vi "PH_Beamline.Calc Booster State.vi"(0 "i ref in":refnum<vi>, 2 "PA Exit closed or shining into LL":bool, 5 "error in (no error)":errorcluster) -> (14 "i ref out":refnum<vi>, 16 "Not shining to Mirrortower":bool, 17 "Not shining Experiment LB":bool, 19 "error out":errorcluster)   [LabVIEW 2014, in "PH_Beamline.lvlib"]
doc: "This VI calculates the Booster state of the Beamline."
uses:
  PH_Beamline.lvlib
  PH_Common/PH_Common.lvlib
  PH_BL-Master/PH_BL-Master.lvlib
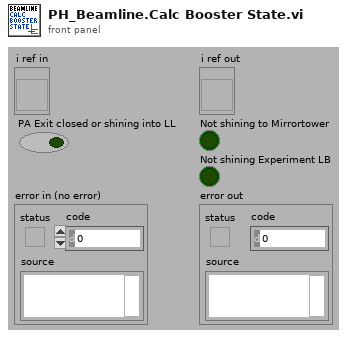
[diagram p1: front panel]
types:
  T1 = typedef "PH_Beamline.lvlib/PH_Beamline.i attribute.ctl" = cluster{"GUI Refs":cluster{"PA ok":refnum<vi>, "MA ok":refnum<vi>, "fs FE ok":refnum<vi>, "ns FE ok":refnum<vi>, "PA ED ok":refnum<vi>, "MAS ok":refnum<vi>, "Booster ok":refnum<vi>, "Mirrortower ok":refnum<vi>, "In.-Box ok":refnum<vi>, "Compressor ok":refnum<vi>, "Experiment LB ok":refnum<vi>, "Experiment LL ok":refnum<vi>, "PHELIX_Beckhoff_Watchdog":refnum<vi>, "Shutters closed":refnum<vi>, "uOPA ok":refnum<vi>, "Vacuum no shotcond Comp LB":refnum<vi>}, "Refs BL MA":refnum<vi>[], "Refs BL MA-IB":refnum<vi>[], "Refs BL fs":refnum<vi>[], "Refs BL PA ED":refnum<vi>[], "Refs BL MAS":refnum<vi>[], "Refs BL Boo":refnum<vi>[], "Refs BL ns":refnum<vi>[], "Refs BL Mirrortower":refnum<vi>[], "Refs BL Compressor":refnum<vi>[], "Refs BL Exp LB":refnum<vi>[], "Radiation Safety":cluster{"Exp Laserbay":cluster{"Ref Op Mode":refnum<vi>, "Ref Laserbay evacuated":refnum<vi>, "Tagname LB evacuated":string, "Shot Mode":T2, "Laserbay evacuated?":i32, "Tagname HV room locked":string, "HV room locked?":i32, "Ref HV room locked":refnum<vi>, "Tagname bridged?":string, "Ref Bridge":refnum<vi>, "I<1E18W/cm²":bool}, "Exp Laserlab":cluster{"Ref Op Mode":refnum<vi>, "Ref Laserlab evacuated":refnum<vi>, "Tagname LL evacuated":string, "Shot Mode":T2, "Laserlab evacuated?":i32, "Tagname bridged?":string, "Ref Bridge":refnum<vi>, "I<1E18W/cm²":bool}}, "Refs BL LL":refnum<vi>[], "PP Igni Heating GUI Refs":refnum<vi>[], "PP Igni Heating Tagnames ":string[], "Refs BL PA":cluster{"undelayed Line before Shutter":refnum<vi>[], "undelayed Line after Shutter":refnum<vi>[], "before Bypass":refnum<vi>[], "delayed Line before Shutter":refnum<vi>[], "delayed Line after Shutter":refnum<vi>[], "before Shutter Input":refnum<vi>[], "after Shutter Input":refnum<vi>[], "Bypass":refnum<vi>[], "before Shutter Exit":refnum<vi>[], "after Shutter Exit":refnum<vi>[], "to MA":refnum<vi>[], "to Lab":refnum<vi>[]}, "BL":cluster{"YLF_BL_Status":i32, "fs_BL_Status":i32, "fs_YLF_BL_Status":i32, "ns_BL_Status":i32, "PA_Input_BL_Status":i32, "PA_UnDelay_BL_Status":i32, "PA_Delay_BL_Status":i32, "PA_BL_Status":i32, "PA_Bypass_BL_Status":i32, "PA_Exit_BL_Status":i32, "PA_LL_BL_Status":i32, "LL_BL_Status":i32, "PA_MA_BL_Status":i32, "MA_Exit_BL_Status":i32, "MA_Z6_BL_Status":i32, "Z6_BL_Status":i32, "MA_LB_BL_Status":i32, "LB_TB2_BL_Status":i32, "PA_before_Bypass_BL_Status":i32, "LB_TB3_BL_Status":i32}, "State Subsystems":cluster{"PA":bool, "MA":bool, "ns FE":bool, "fs FE":bool, "PA ED":bool, "In.-Box":bool, "MAS":bool, "Booster":bool, "Mirrortower":bool, "Compressor":bool, "Experiment LB":bool, "Experiment LL":bool, "uOPA":bool}, "Status Subscriber Information":T3, "Refs BL uOPA":refnum<vi>[], "PA_Input_2_Beam_6PWpGUI not linked?":bool, "PA_Input_Delay_6PGUI not linked?":bool, "Settings":T6}
  T2 = typedef "PH_Beamline.lvlib/PH_Beamline.Operation Mode.ctl" = i32
  T3 = typedef "PH_Beamline.lvlib/PH_Beamline.Status Subscriber Information.ctl" = cluster{"fs Swich YLF":T4, "fs Exit Shutter":T4, "ns Exit Shutter":T4, "PA Input Shutter":T4, "PA PC WP":T4, "PA PC WP 2":T4, "PA Bypass In":T4, "PA Bypass Out":T4, "PA CH 1":T4, "PA delayed":T4, "PA non delayed":T4, "PA Exit Shutter":T4, "PA Switch Lab":T4, "PA Bridge CH Input MA":T4, "MA Diffusor IB":T4, "MA IB Ready":T4, "MA CH 1":T4, "MA CH 2":T4, "MA CH 3":T4, "MA CH 4":T4, "MA Shutter Align Cam":T4, "MA Position MM5":T4, "Calorimeter Switch":T4, "BL Z6 CH 9":T4, "BL Z6 Beamdump":T4, "BL Z6 Shutter":T4, "COS Sensitivity Switch":T4, "Exp LB Shutter":T4, "Exp LB TB 2":T4, "Exp LB TB 3":T4, "PA LL Input CH":T4, "PA LL Output CH":T4, "LL Comp Input Shutter":T4, "LL Comp Output Shutter":T4, "LL Comp FF Shutter":T4, "Exp LL Shutter":T4, "MA IM In IB":T4, "MA IM Out IB":T4, "MA DB In IB":T4, "MA DB Out IB":T4, "Exp LB Shutter Interlock":T4, "Exp LL Shutter Interlock":T4, "MM1 Force Sensor":T4}
  T4 = typedef "PH_BL-Master.lvlib/PH_BL-Master.Status Subscriber Information.ctl" = cluster{"Index of element":i32, "Attributeset":T5}
  T5 = typedef "PH_BL-Master.lvlib/PH_BL-Master.Attribute Set.ctl" = enum16{"Boolean Status Service Subscriber", "Picture Status Service Subscriber"}
  T6 = typedef "PH_Beamline_Chief.lvlib/PH_Beamline_Chief.Settings.ctl" = cluster{"PA Doublepass Mode":bool, "Compressor Vaccuum LB not relevant":bool, "Windowshutter TB2 not relevant":bool, "Windowshutter TB3 not relevant":bool}
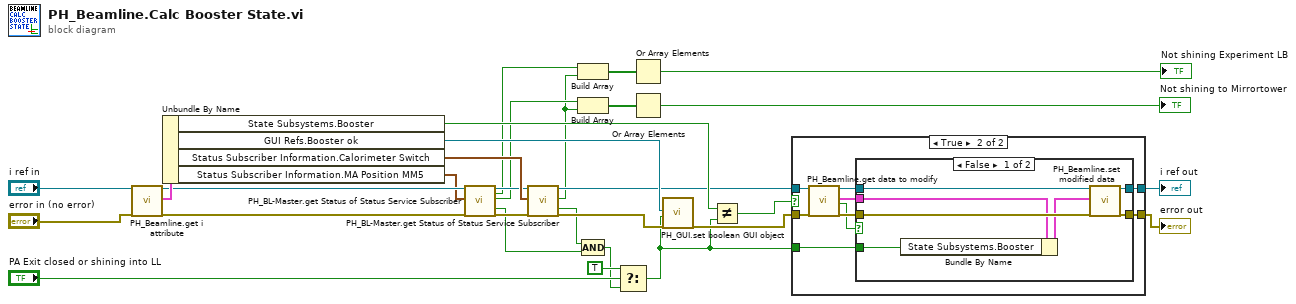
[diagram p0: block diagram]
diagram:
  n1 = call "PH_Beamline.get i attribute.vi"("i ref in"="i ref in", "error in (no error)"="error in (no error)") -> ("i ref out"=w19:refnum<vi>, "i attribute"=w28:T1, "error out"=w18:errorcluster)  [unwired: 15 in]
  n2 = Unbundle By Name(w28) -> ("State Subsystems.Booster"=w26:bool, "GUI Refs.Booster ok"=w29:refnum<vi>, "Status Subscriber Information.Calorimeter Switch"=w17:T4, "Status Subscriber Information.MA Position MM5"=w16:T4)
  n3 = call "PH_BL-Master.get Status of Status Service Subscriber.vi"("i ref in"=w19, "Wanted Status Subscriber Information"=w16, "error in (no error)"=w18) -> ("i ref out"=w15:refnum<vi>, "off/false/out?"=w4:bool, "on/true/in?"=w6:bool, "off/false/out or on/true/in?"=w13:bool, "error out"=w14:errorcluster)  [unwired: 11 in, 1 out]
  n4 = call "PH_BL-Master.get Status of Status Service Subscriber.vi"("i ref in"=w15, "Wanted Status Subscriber Information"=w17, "error in (no error)"=w14) -> ("i ref out"=w25:refnum<vi>, "on/true/in?"=w3:bool, "off/false/out or on/true/in?"=w12:bool, "error out"=w30:errorcluster)  [unwired: 11 in, 2 out]
  n5 = Build Array(w4, w3) -> (w2:bool[])
  n6 = Build Array(w6, w3) -> (w7:bool[])
  n7 = Compound Arithmetic op=AND(w12, w13) -> (w9:bool)
  n8 = Select(t=TRUE, s="PA Exit closed or shining into LL", f=w9) -> (s? t:f=w8:bool)
  n9 = Or Array Elements(Boolean array=w2) -> (logical OR=→"Not shining Experiment LB":bool)
  n10 = Or Array Elements(Boolean array=w7) -> (logical OR=→"Not shining to Mirrortower":bool)
  n11 = call "PH_GUI.set boolean GUI object.vi"("Boolean Knob GUI Ref"=w29, "Value"=w8, "error in (no error)"=w30) -> ("error out"=w23:errorcluster)  [unwired: 16 in]
  n12 = Not Equal?(x=w26, y=w8) -> (x != y?=w27:bool)
  n13 = case shown="True" w27 {
    tunnel: [w32 w37] -> w24
    tunnel: [w31 w36] -> w22
    tunnel: w8 -> [_ w35]
    tunnel: w23 -> [w31 w34]
    tunnel: w25 -> [w32 w33]
    frame False {
    }
    frame True {
      n14 = call "PH_Beamline.get data to modify.vi"("i ref in"=w33, "error in (no error)"=w34) -> ("i ref out"=w40:refnum<vi>, "i attribute"=w38:T1, "timed out"=w39:bool, "error out"=w41:errorcluster)  [unwired: 14 in]
      n15 = case shown="False" w39 {
        tunnel: w41 -> [w48 w49]
        tunnel: w40 -> [w47 w50]
        tunnel: [w46 w49] -> w36
        tunnel: [w45 w50] -> w37
        tunnel: w38 -> [w44 _]
        tunnel: w35 -> [w42 _]
        frame False {
          n16 = Bundle By Name(cluster=w44, "State Subsystems.Booster"=w42) -> (w43:T1)
          n17 = call "PH_Beamline.set modified data.vi"("i ref in"=w47, "i attribute"=w43, "error in (no error)"=w48) -> ("i ref out"=w45:refnum<vi>, "error out"=w46:errorcluster)  [unwired: 15 in]
        }
        frame True {
        }
      }
    }
  }
  "i ref out" <- w24
  "error out" <- w22
